vi "Set-last-activity.vi"(8 "error in (no error)":errorcluster, 9 "Last contact":dbl, 10 "Client index":i32, 11 "ModComm in":T1) -> (0 "error out":errorcluster, 3 "ModComm out":T1)   [LabVIEW 2013, in "SLMServer.lvlib" / "SLMServer.lvclass"]
uses:
  SLMServer.lvclass
  Object-reference.ctl
  SLMServer.lvclass/SLMServer.ctl
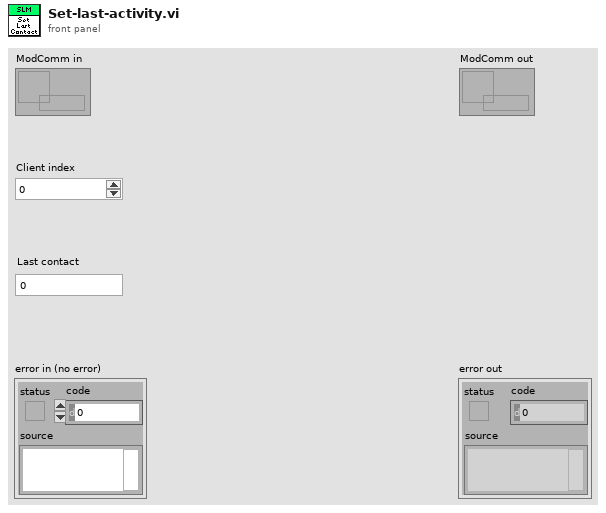
[diagram p1: front panel]
types:
  T1 = typedef "SLMServer.lvlib/SLMServer.lvclass/Object-reference.ctl" = refnum<data-value>
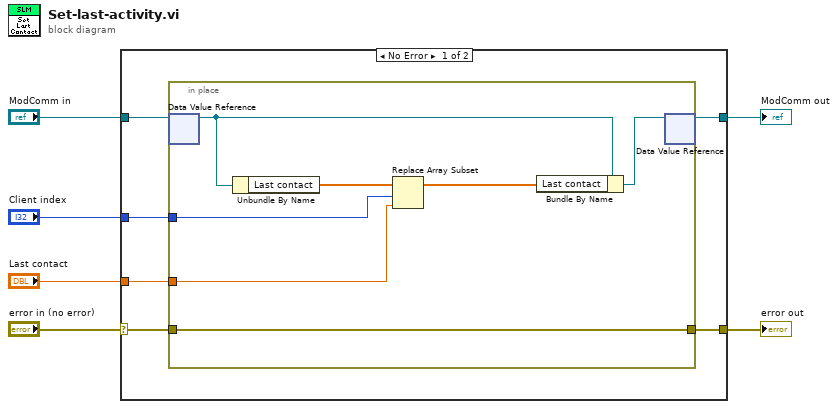
[diagram p0: block diagram]
diagram:
  n1 = case shown="No Error" "error in (no error)" {
    selector: "error in (no error)" -> [w12 w21]
    tunnel: [w8 w21] -> w5
    tunnel: [w7 w20] -> w3
    tunnel: "ModComm in" -> [w11 w20]
    tunnel: "Client index" -> [w10 _]
    tunnel: "Last contact" -> [w9 _]
    frame No Error {
      n2 = in-place {
        in-place-border: w12 -> [w16]
        in-place-border: w10 -> [w18]
        in-place-border: w9 -> [w17]
        in-place-border: [w16] -> w8
        n3 = in-place-dvr #1(w11) -> (w14:refnum<class "SLMServer.lvclass">)  [unwired: 1 out]
        n4 = Unbundle By Name(w14) -> ("Last contact"=w19:dbl[])
        n5 = Replace Array Subset(array=w19, new element=w17, index=w18) -> (w15:dbl[])
        n6 = Bundle By Name(cluster=w14, "Last contact"=w15) -> (w13:refnum<class "SLMServer.lvclass">)
        n7 = in-place-dvr #1(w13) -> (w7:T1)  [unwired: 1 out]
      }
    }
    frame Error {
    }
  }
  "error out" <- w5
  "ModComm out" <- w3
